vi "Send Message Modules.vi"(5 "All Modules":bool, 7 "priority (normal)":T1, 8 "Error In":errorcluster, 9 "Data":variant, 10 "Message":string, 11 "Target ModuleName In":T2[](array[typedef])) -> (0 "error in (no error)":errorcluster)   [LabVIEW 2021, in "Architecture.lvlib"]
doc: "This method is used to send an asynchronous message to a target module. It generates a user event that will be handled by target module's event structure."
uses:
  Architecture.lvlib
  Typedefs/Enum_Module_Name.ctl
  <vilib>/event_ctls.llb/usereventprio.ctl
  Typedefs/Message.ctl
  Typedefs/Module References.ctl
  Typedefs/FGV Ref. Modules Function.ctl
  Modules/Configuration/Configuration.lvlib
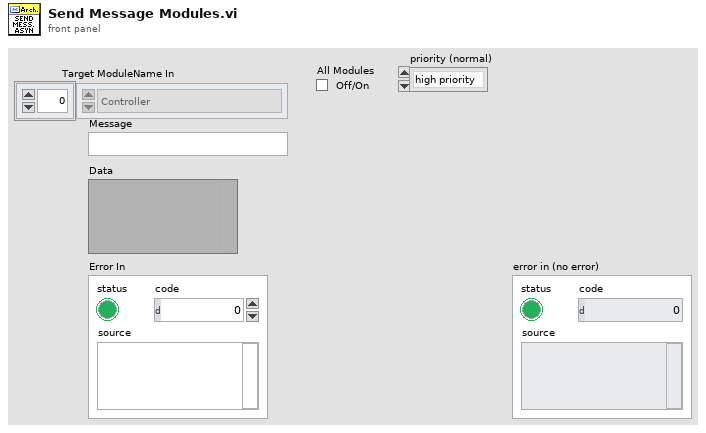
[diagram p1: front panel]
types:
  T1 = typedef "usereventprio.ctl" = enum32{"high priority", "normal priority"}
  T2 = typedef "Configuration.lvlib/Enum_Module_Name.ctl" = enum16{"Configuration", "Error_Handler", "Log", "Database", "Controller", "UI Module", "Sound Manager"}
  T3 = typedef "Architecture.lvlib/Message.ctl" = cluster{"Message":string, "Data":variant, "syn":bool}
  T4 = typedef "Architecture.lvlib/FGV Ref. Modules Function.ctl" = enum16{"Init ", "Add Module", "Get Module", "Get All", "Add Asynchronous Run Ref", "Dispose"}
  T5 = typedef "Architecture.lvlib/Module References.ctl" = cluster{"ModuleName":T2, "Queue":refnum<queue>, "user event":refnum<user-event>, "VI Refnum":refnum<vi>, "ShowFP":bool, "StatesTracking Enabled":bool}
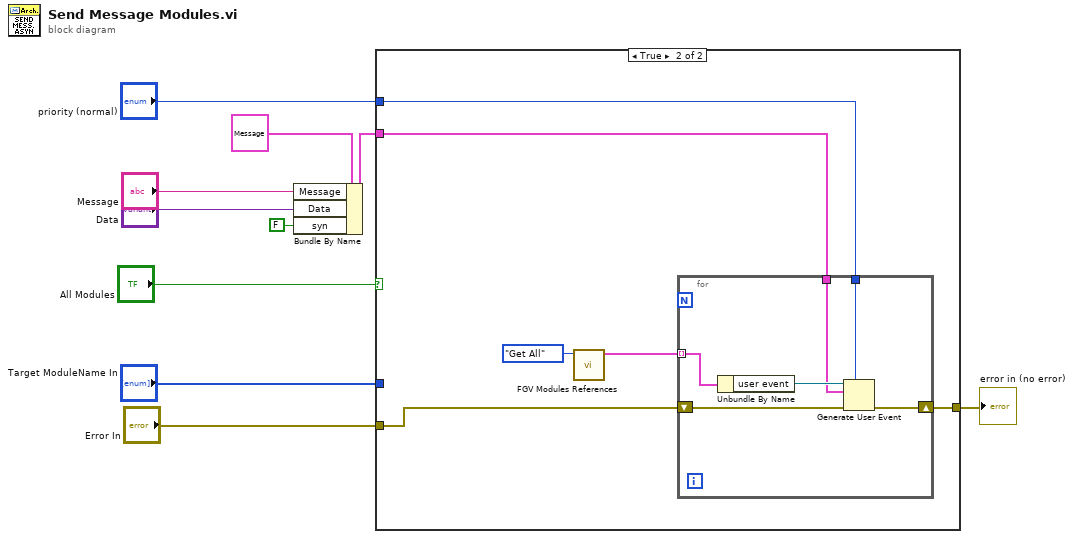
[diagram p0: block diagram]
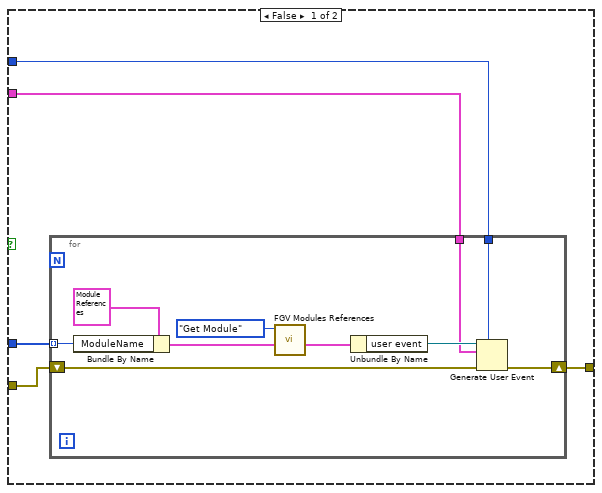
[diagram p2: hidden frame]
diagram:
  n1 = Bundle By Name(cluster=T3 {"Message"="", "Data"=variant, "syn"=FALSE} ("event data"), "Message"="Message", "Data"="Data", "syn"=FALSE) -> (w8:T3)
  n2 = case shown="True" "All Modules" {
    tunnel: "Target ModuleName In" -> [w15 _]
    tunnel: w8 -> [w14 w31]
    tunnel: "priority (normal)" -> [w13 w30]
    tunnel: [w12 w29] -> w4
    tunnel: "Error In" -> [w11 w28]
    frame False {
      n3 = for {
        tunnel: w15 -> [w24] mode=indexing
        tunnel: w14 -> [w19]
        tunnel: w13 -> [w18]
        shift-right: [w17] -> w12
        shift-left: w11 -> [w16]
        n4 = Bundle By Name(cluster=T5 {"ModuleName"=enum."Controller", "Queue"=refnum, "user event"=refnum, "VI Refnum"=refnum, "ShowFP"=FALSE, "StatesTracking Enabled"=FALSE} ("Module_Refs"), "ModuleName"=w24) -> (w23:T5)
        n5 = call "FGV Modules References.vi"("Module_Refs"=w23, "FGV Ref. Function In"=FGV_Ref._Modules_Function."Get Module") -> ("Module_Ref Out"=w21:T5)  [unwired: 6 in, 3 out]
        n6 = Unbundle By Name(w21) -> ("user event"=w20:refnum<user-event>)
        n7 = Generate User Event(priority (normal)=w18, user event=w20, event data cluster=w19, error in=w16) -> (error out=w17:errorcluster)  [unwired: 1 out]
      }
    }
    frame True {
      n8 = call "FGV Modules References.vi"("FGV Ref. Function In"=FGV_Ref._Modules_Function."Get All") -> ("All Modules Refs"=w26:T5[])  [unwired: 7 in, 3 out]
      n9 = for {
        tunnel: w31 -> [w36]
        tunnel: w30 -> [w35]
        shift-right: [w34] -> w29
        shift-left: w28 -> [w33]
        tunnel: w26 -> [w32] mode=indexing
        n10 = Unbundle By Name(w32) -> ("user event"=w37:refnum<user-event>)
        n11 = Generate User Event(priority (normal)=w35, user event=w37, event data cluster=w36, error in=w33) -> (error out=w34:errorcluster)  [unwired: 1 out]
      }
    }
  }
  "error in (no error)" <- w4
